vi "LVClass_WavefrontCorrector Get Temporization.vi"(0 "WavefrontCorrector in":refnum<class "WavefrontCorrector.lvclass">, 11 "error in (no error)":errorcluster) -> (4 "WavefrontCorrector out":refnum<class "WavefrontCorrector.lvclass">, 6 "Sleep after command apply (ms)":i32, 15 "error out":errorcluster)   [LabVIEW 2020, in "WavefrontCorrector.lvclass"]
doc: "Get current WavefrontCorrector preference \"Time to stabilization (ms)\".\n\n<B>correctorIn</B> : WavefrontCorrector object.\n<B>correctorOut</B> : WavefrontCorrector object.\n<B>sleep_after_movement</B> : WavefrontCorrector preferences : Time to stabilization (ms)."
uses:
  WavefrontCorrector.lvclass
  WavefrontCorrector.lvclass/WavefrontCorrector.ctl
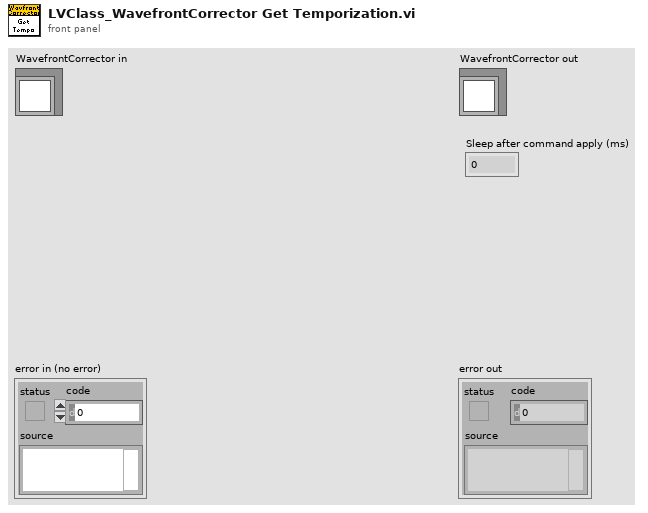
[diagram p1: front panel]
types:
  T1 = typedef "ClassID.ctl" = i64
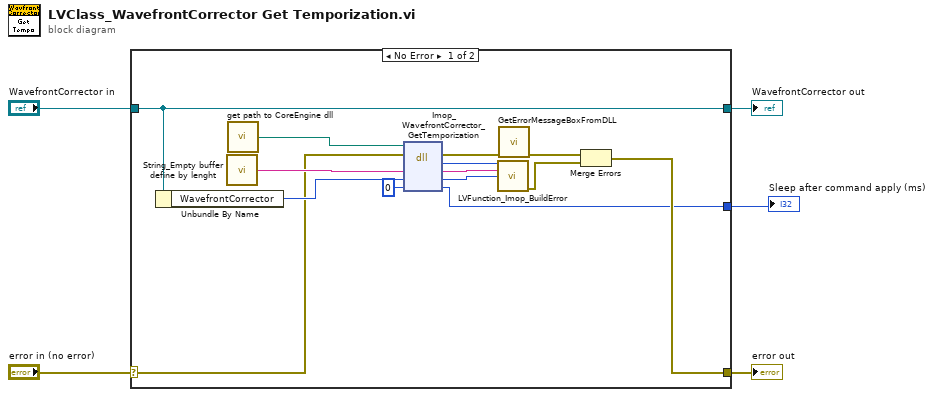
[diagram p0: block diagram]
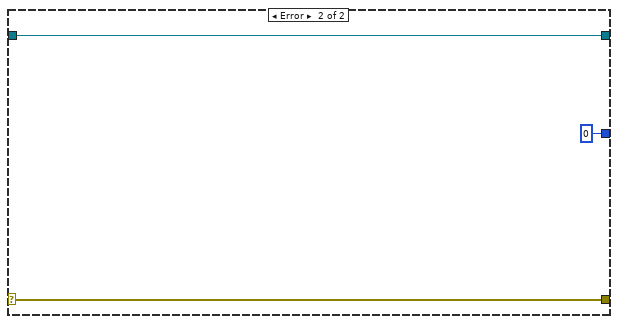
[diagram p2: hidden frame]
diagram:
  n1 = case shown="No Error" "error in (no error)" {
    selector: "error in (no error)" -> [w7 w22]
    tunnel: [w11 w22] -> w4
    tunnel: [w19 w21] -> w2
    tunnel: "WavefrontCorrector in" -> [w19 w21]
    tunnel: [w10 0 ("sleep_after_movement")] -> w1
    frame No Error {
      n2 = Unbundle By Name(w19) -> ("WavefrontCorrector"=w17:T1)
      n3 = call "String_Empty buffer define by lenght.vi"() -> ("Empty buffer"=w16:string)  [unwired: 1 in]
      n4 = call "get path to CoreEngine dll.vi"() -> ("path to wavekit library"=w18:path)  [unwired: 14 in, 1 out]
      n5 = dll-call lib="D:/FLE/0.Code/CoreEngine4_Suite/LV2011_interface/DLLs/c_interface_vc100.dll" fn="Imop_WavefrontCorrector_GetTemporization"(path in=w18, error in=w7, "message"=w16, "Wavefront Corrector"=w17, "Sleep after movement"=0) -> (error out=w9:errorcluster, "return type"=w14:i32, "message"=w13:string, "Wavefront Corrector"=w6:i64, "Sleep after movement"=w10:i32)  [unwired: 1 in, 1 out]
      n6 = call "LVFunction_Imop_BuildError.vi"("code"=w14, "String to Prepend to source (\"\")"=w13, "Adresse"=w6) -> ("error out"=w12:errorcluster)  [unwired: 12 in]
      n7 = call "GetErrorMessageBoxFromDLL.vi"("error IN"=w9) -> ("error OUT"=w8:errorcluster)  [unwired: 10 in]
      n8 = Merge Errors(w8, w12) -> (w11:errorcluster)
    }
    frame Error {
    }
  }
  "error out" <- w4
  "WavefrontCorrector out" <- w2
  "Sleep after command apply (ms)" <- w1
